vi "Main.vi"() -> ()   [LabVIEW 2015]
uses:
  <vilib>/myRIO/Instrument Drivers/Onboard IO/PWM/typedefs/PWM Reference.ctl
  <vilib>/myRIO/Common/Instrument Driver Framework/Utilities/typedefs/myRIO Generic Hardware Reference.ctl
  <vilib>/myRIO/Common/Instrument Driver Framework/Utilities/typedefs/Hardware Version Enum.ctl
  <vilib>/myRIO/Common/Instrument Driver Framework/Utilities/typedefs/myRIO v1.0 Reference.ctl
  <vilib>/myRIO/Common/Instrument Driver Framework/Utilities/typedefs/Generic FPGA Reference.ctl
  <vilib>/myRIO/Common/Instrument Driver Framework/myRIO v1.0/PWM/typedefs/PWM Channels Enum.ctl
  <vilib>/myRIO/Instrument Drivers/Onboard IO/PWM/typedefs/PWM Configuration.ctl
  <vilib>/userdefined/High Color/nirio_resource_hc.ctl
  <vilib>/myRIO/Instrument Drivers/Onboard IO/DIO/typedefs/DIO Reference.ctl
  <vilib>/myRIO/Common/Instrument Driver Framework/myRIO v1.0/DIO/typedefs/DIO Channels List.ctl
  <vilib>/myRIO/Common/Instrument Driver Framework/myRIO v1.0/DIO/typedefs/DIO Channels Enum.ctl
  <vilib>/myRIO/Common/Instrument Driver Framework/Utilities/vis/Is FPGA Ref Available.vi
  <vilib>/myRIO/Common/Instrument Driver Framework/myRIO v1.0/DIO/vis/myRIO v1.1 Open DIO.vi
  <vilib>/myRIO/Instrument Drivers/Onboard IO/DIO/vis/Write.vi
  <vilib>/myRIO/Common/Instrument Driver Framework/myRIO v1.0/PWM/vis/myRIO v1.1 Open PWM.vi
  <vilib>/myRIO/Common/Instrument Driver Framework/Utilities/vis/Validate Channels.vi
  <vilib>/myRIO/Common/Instrument Driver Framework/myRIO v1.0/DIO/vis/myRIO v1.0 Reserve DIO.vi
  <vilib>/myRIO/Common/Instrument Driver Framework/myRIO v1.0/PWM/vis/myRIO v1.0 Reserve PWM.vi
  <vilib>/myRIO/Instrument Drivers/Onboard IO/PWM/vis/Set Duty Cycle and Frequency.vi
  <vilib>/myRIO/Common/Instrument Driver Framework/myRIO v1.0/PWM/vis/myRIO v1.0 Close PWM.vi
  <vilib>/myRIO/Common/Instrument Driver Framework/myRIO v1.0/UART/vis/myRIO v1.0 Close UART.vi
  <vilib>/myRIO/Common/Instrument Driver Framework/myRIO v1.0/Resource Manager/vis/myRIO v1.0 Reserve Channel List.vi
  <vilib>/myRIO/Common/Instrument Driver Framework/myRIO v1.0/DIO/vis/myRIO v1.0 Build MUX Configuration DIO.vi
  <vilib>/myRIO/Common/Instrument Driver Framework/myRIO v1.0/PWM/vis/myRIO v1.0 Build MUX Configuration PWM.vi
  <vilib>/myRIO/Common/Instrument Driver Framework/myRIO v1.0/PWM/vis/myRIO v1.0 Unreserve PWM.vi
  <vilib>/myRIO/Common/Instrument Driver Framework/myRIO v1.0/Resource Manager/vis/myRIO v1.0 Reserve Channel.vi
  <vilib>/myRIO/Common/Instrument Driver Framework/myRIO v1.0/Resource Manager/vis/myRIO v1.0 Unreserve Channel.vi
  <vilib>/myRIO/Common/Instrument Driver Framework/myRIO v1.0/Resource Manager/vis/myRIO v1.0 Create Configuration List.vi
  <vilib>/myRIO/Common/Instrument Driver Framework/myRIO v1.0/Resource Manager/vis/myRIO v1.0 Unreserve Channel List.vi
  <vilib>/myRIO/Common/Instrument Driver Framework/myRIO v1.0/Resource Manager/vis/myRIO v1.0 Build Mutex Name.vi
  <vilib>/Utility/VariantDataType/GetNumericInfo.vi
  <vilib>/Utility/error.llb/Error Cluster From Error Code.vi
  <vilib>/myRIO/Common/Instrument Driver Framework/myRIO v1.0/myRIO v1.1 Open.vi
  <vilib>/myRIO/Common/Instrument Driver Framework/Utilities/vis/IO Manager.vi
  <vilib>/myRIO/Common/Instrument Driver Framework/Utilities/vis/Configuration Manager.vi
  <vilib>/myRIO/Common/Instrument Driver Framework/myRIO v1.0/Resource Manager/vis/myRIO v1.0 Configure IO.vi
  <vilib>/myRIO/Common/Instrument Driver Framework/myRIO v1.0/myRIO v1.0 Close.vi
  <vilib>/myRIO/Common/Instrument Driver Framework/myRIO v1.0/PWM/vis/myRIO v1.0 Write PWM.vi
  <vilib>/myRIO/Common/Instrument Driver Framework/myRIO v1.0/PWM/vis/myRIO v1.0 Shutdown PWM.vi
  <vilib>/myRIO/Common/Instrument Driver Framework/Utilities/vis/FPGA Ref Manager.vi
  <vilib>/myRIO/Common/Instrument Driver Framework/myRIO v1.0/myRIO v1.0 Reset FPGA.vi
  <vilib>/myRIO/Common/Instrument Driver Framework/myRIO v1.0/IRQ/vis/myRIO v1.0 IRQ Info FGV.vi
  <vilib>/myRIO/Common/Instrument Driver Framework/myRIO v1.0/IRQ/vis/myRIO v1.0 Timer IRQ Info FGV.vi
  <vilib>/myRIO/Common/Instrument Driver Framework/myRIO v1.0/IRQ/vis/myRIO v1.0 ISR Agent.vi
  <vilib>/myRIO/Common/Instrument Driver Framework/myRIO v1.0/DIO/vis/myRIO v1.0 Write DIO.vi
  <vilib>/myRIO/Instrument Drivers/Onboard IO/PWM/vis/myRIO PWM Open.xnode
  <vilib>/myRIO/Express VI/Onboard Devices/LED/LED Express VI.xnode
  <vilib>/myRIO/Instrument Drivers/Onboard IO/DIO/vis/myRIO DIO Open.xnode
  <vilib>/myRIO/Instrument Drivers/Onboard IO/PWM/PWM.lvlib
  <vilib>/myRIO/Instrument Drivers/Utilities/Utilities.lvlib
  <vilib>/myRIO/Instrument Drivers/Onboard IO/DIO/DIO.lvlib
panel:
  in  "Water Spill Guard":bool
  out "Sensor Pin":T1
  out "Gripper Pin":T1
  out "Pour Pin":T1
  in  "Pour":bool
  out "Information":string="Pour"
  out "Counter":dbl=1.0
  out "New Duty Cycle":dbl=nan
  in  "Stop [ESC]":bool
  in  "Gripper":bool
  out "Water Detected":bool
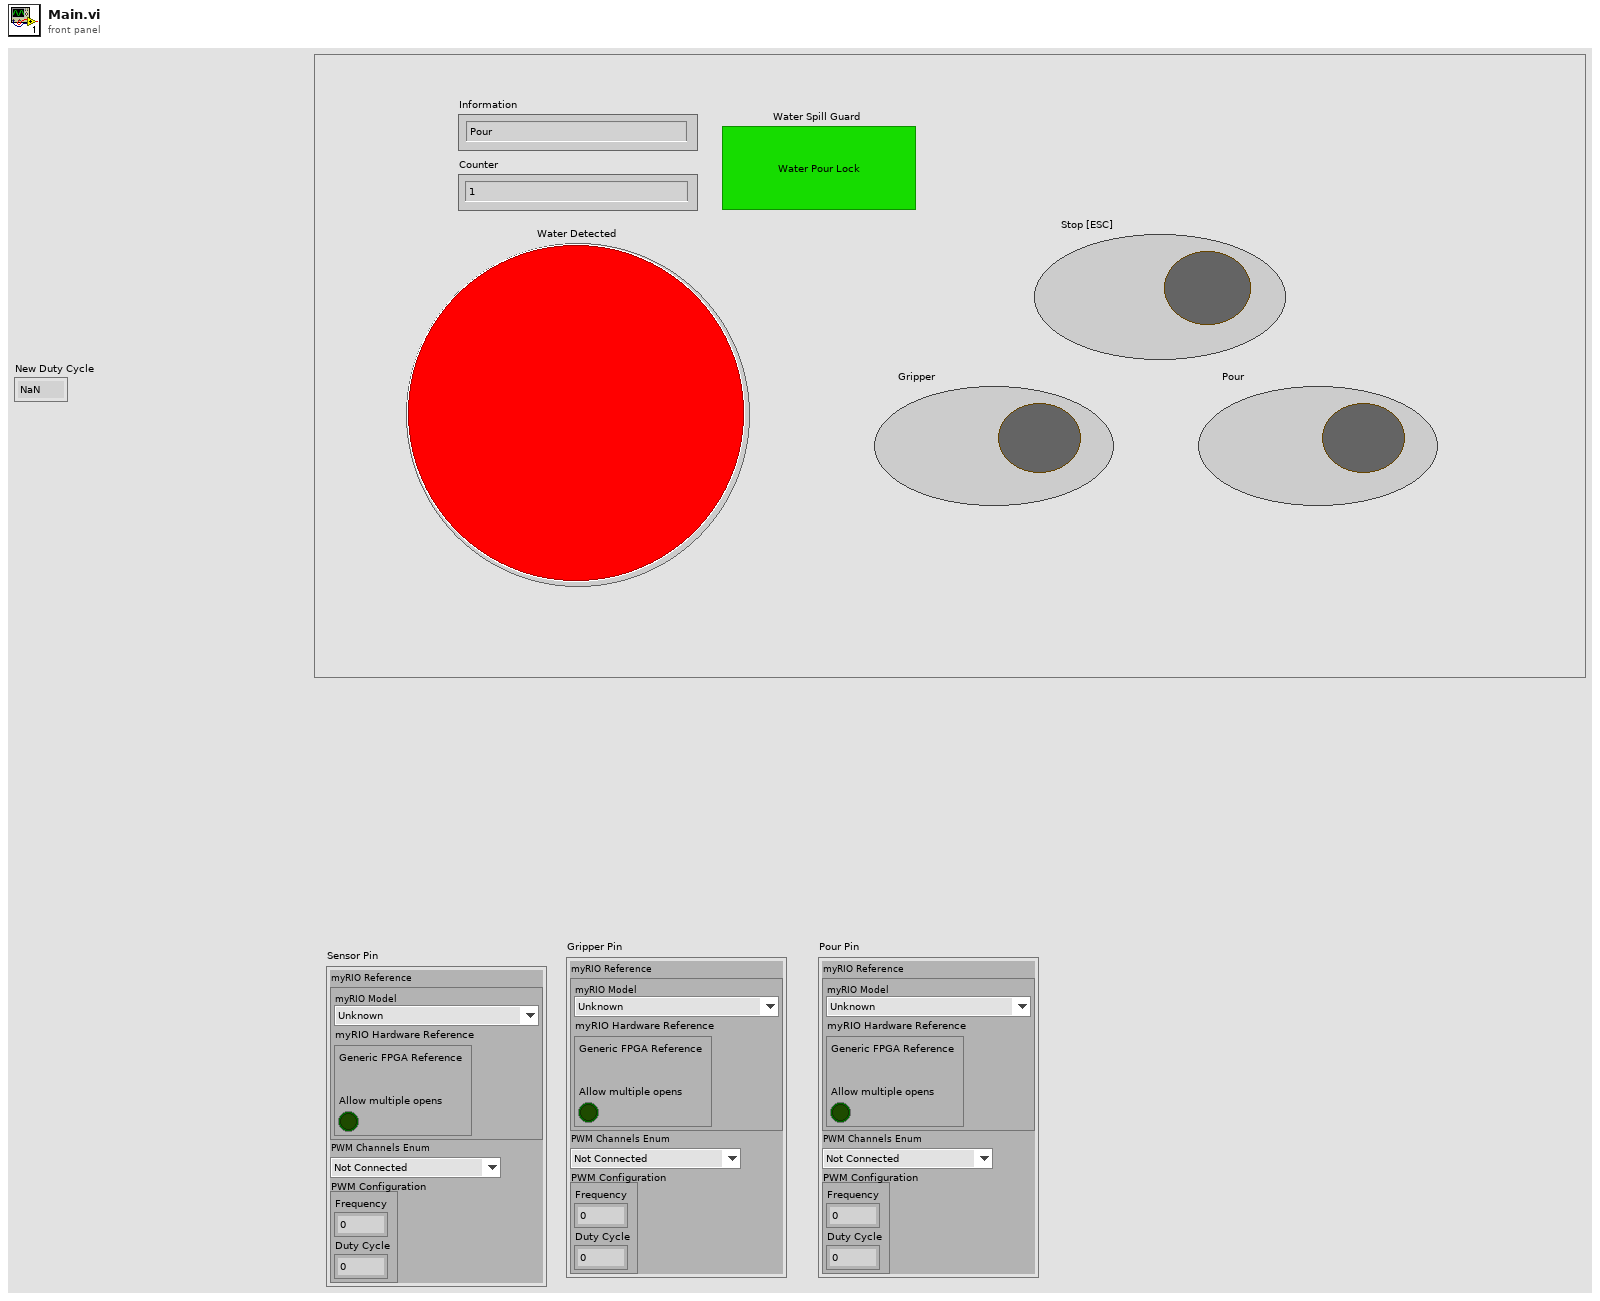
[diagram p1: front panel]
types:
  T1 = typedef "PWM.lvlib/PWM Reference.ctl" = cluster{"myRIO Reference":T2, "PWM Channels Enum":T6, "PWM Configuration":T7}
  T2 = typedef "myRIO Generic Hardware Reference.ctl" = cluster{"myRIO Model":T3, "myRIO Hardware Reference":T4}
  T3 = typedef "Hardware Version Enum.ctl" = enum16{"Unknown", "myRIO-1900", "myRIO-1950", "roboRIO"}
  T4 = typedef "myRIO v1.0 Reference.ctl" = cluster{"Generic FPGA Reference":T5, "Allow multiple opens":bool}
  T5 = typedef "Generic FPGA Reference.ctl" = refnum<k20>
  T6 = typedef "PWM Channels Enum.ctl" = enum16{"Not Connected", "C/PWM0", "C/PWM1", "A/PWM0", "A/PWM1", "A/PWM2", "B/PWM0", "B/PWM1", "B/PWM2", "PWM/PWM0", "PWM/PWM1", "PWM/PWM2", "PWM/PWM3", "PWM/PWM4", "PWM/PWM5", "PWM/PWM6", "PWM/PWM7", "PWM/PWM8", "PWM/PWM9"}
  T7 = typedef "PWM.lvlib/PWM Configuration.ctl" = cluster{"Frequency":dbl, "Duty Cycle":dbl}
  T8 = typedef "nirio_resource_hc.ctl" = tag
  T9 = typedef "DIO.lvlib/DIO Reference.ctl" = cluster{"myRIO Reference":T2, "DIO Channels List":T10}
  T10 = typedef "DIO Channels List.ctl" = T11[]
  T11 = typedef "DIO Channels Enum.ctl" = enum16{"Not Connected", "C/DIO0", "C/DIO1", "C/DIO2", "C/DIO3", "C/DIO4", "C/DIO5", "C/DIO6", "C/DIO7", "A/DIO0", "A/DIO1", "A/DIO2", "A/DIO3", "A/DIO4", "A/DIO5", "A/DIO6", "A/DIO7", "A/DIO8", "A/DIO9", "A/DIO10", "A/DIO11", "A/DIO12", "A/DIO13", "A/DIO14", "A/DIO15", "B/DIO0", "B/DIO1", "B/DIO2", "B/DIO3", "B/DIO4", "B/DIO5", "B/DIO6", "B/DIO7", "B/DIO8", "B/DIO9", "B/DIO10", "B/DIO11", "B/DIO12", "B/DIO13", "B/DIO14", "B/DIO15", "LED0", "LED1", "LED2", "LED3", "Button0", "DIO/DIO0", "DIO/DIO1", "DIO/DIO2", "DIO/DIO3", "DIO/DIO4", "DIO/DIO5", "DIO/DIO6", "DIO/DIO7", "DIO/DIO8", "DIO/DIO9", "SPI/CS0", "SPI/CS1", "SPI/CS2", "SPI/CS3", "LED RADIO (Green)", "LED RADIO (Red)", "LED COMM (Green)", "LED COMM (Red)", "LED MODE (Green)", "LED MODE (Red)"}
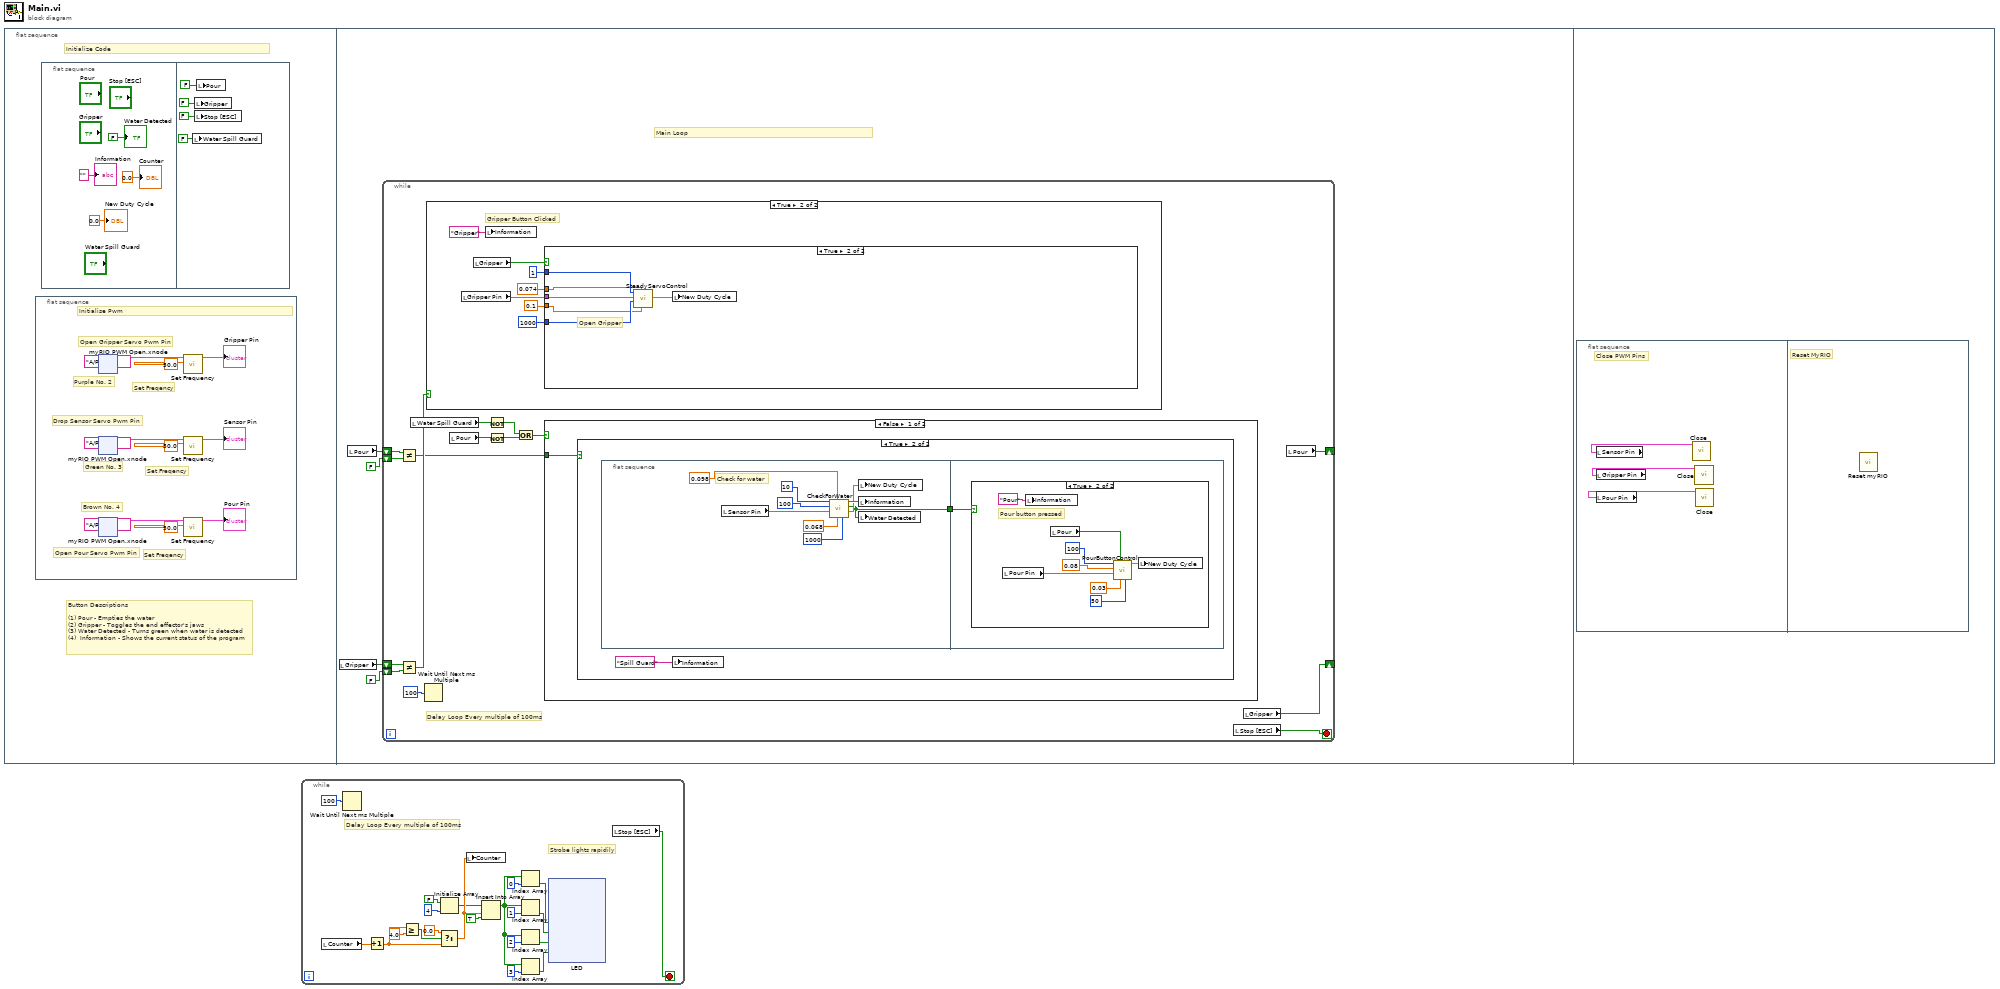
[diagram p0: block diagram]
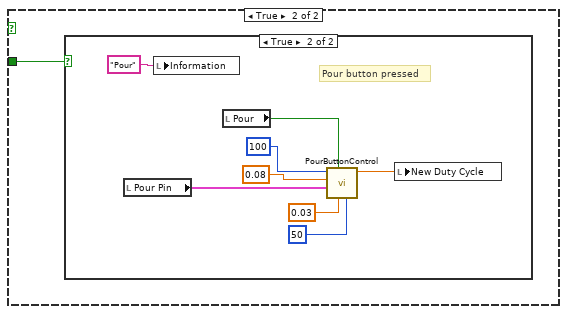
[diagram p4: hidden frame]
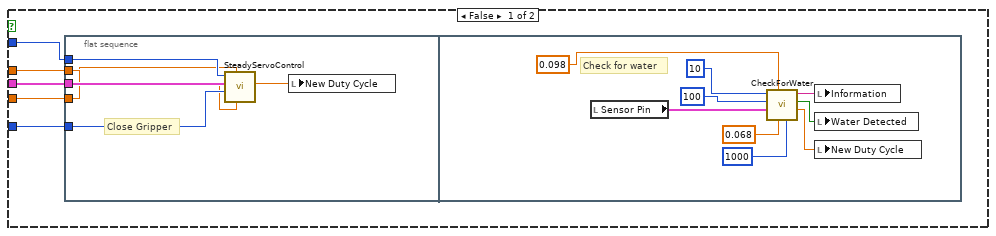
[diagram p7: hidden frame]
diagram:
  n1 = flat-sequence {
    frame #0 {
      # "Button Descriptions\n\n(1) Pour - Empties the water\n(2) Gripper - Toggles the end effector's jaws\n(3) Water Detected - Turns green when water is detected\n(4)  Information - Shows the current status of the program"
      # "Initialize Code"
      n2 = flat-sequence {
        frame #0 {
          # "Green No. 3"
          # "Set Freqency"
          # "Drop Sensor Servo Pwm Pin"
          # "Initialise Pwm"
          # "Purple No. 2"
          # "Set Freqency"
          # "Open Gripper Servo Pwm Pin"
          # "Set Freqency"
          # "Brown No. 4"
          # "Open Pour Servo Pwm Pin"
          n3 = xnode "myRIO PWM Open.xnode"("Channel Name"=tag "A/PWM2") -> ("PWM Ref Out"=w7:T1)  [unwired: 2 in, 1 out]
          n4 = xnode "myRIO PWM Open.xnode"("Channel Name"=tag "A/PWM1") -> ("PWM Ref Out"=w2:T1)  [unwired: 2 in, 1 out]
          n5 = xnode "myRIO PWM Open.xnode"("Channel Name"=tag "A/PWM0") -> ("PWM Ref Out"=w10:T1)  [unwired: 2 in, 1 out]
          n6 = call <vilib>:"Set Frequency.vi"("Frequency [Hz]"=50.0, "PWM Ref In"=w7) -> ("PWM Ref Out"=→"Gripper Pin":T1)  [unwired: 7 in, 1 out]
          n7 = call <vilib>:"Set Frequency.vi"("Frequency [Hz]"=50.0, "PWM Ref In"=w2) -> ("PWM Ref Out"=→"Sensor Pin":T1)  [unwired: 7 in, 1 out]
          n8 = call <vilib>:"Set Frequency.vi"("Frequency [Hz]"=50.0, "PWM Ref In"=w10) -> ("PWM Ref Out"=→"Pour Pin":T1)  [unwired: 7 in, 1 out]
        }
      }
      n9 = flat-sequence {
        frame #0 {
          "Water Detected" <- FALSE ("Water Detected")
          "Counter" <- 0.0 ("Counter")
          "Information" <- "" ("Information")
          "New Duty Cycle" <- 0.0 ("New Duty Cycle")
        }
        frame #1 {
          n10 = local write "Water Spill Guard"(FALSE ("Water Spill Guard")) -> ()
          n11 = local write "Gripper"(FALSE ("Pour")) -> ()
          n12 = local write "Stop [ESC]"(FALSE ("Pour")) -> ()
          n13 = local write "Pour"(FALSE ("Pour")) -> ()
        }
      }
    }
    frame #1 {
      # "Main Loop"
      n14 = local read "Gripper"() -> (w72:bool)
      n15 = local read "Pour"() -> (w70:bool)
      n16 = while {
        shift-right: [w87] -> _
        shift-left: w72 -> [w85]
        shift-left: FALSE ("Gripper") -> [w84]
        shift-right: [w79] -> _
        shift-left: w70 -> [w81]
        shift-left: FALSE ("Pour") -> [w80]
        stop <- w83 stop-if-true
        # "Delay Loop Every multiple of 100ms"
        n17 = Not Equal?(x=w81, y=w80) -> (x != y?=w73:bool)
        n18 = Not Equal?(x=w85, y=w84) -> (x != y?=w86:bool)
        n19 = local read "Water Spill Guard"() -> (w75:bool)
        n20 = Wait Until Next ms Multiple(millisecond multiple=u32 100) -> ()  [unwired: 1 out]
        n21 = case shown="True" w86 {
          frame False {
          }
          frame True {
            # "Gripper Button Clicked"
            n22 = local read "Gripper Pin"() -> (w122:T1)
            n23 = local read "Gripper"() -> (w123:bool)
            n24 = local write "Information"("Gripper" ("Information")) -> ()
            n25 = case shown="True" w123 {
              tunnel: w122 -> [w129 w147]
              tunnel: u32 1 ("Wait Time") -> [w128 w149]
              tunnel: 1000 ("Steps") -> [w127 w148]
              tunnel: 0.074 ("Prev Duty Cycle") -> [w126 w146]
              tunnel: 0.1 ("New Duty Cycle") -> [w125 w145]
              frame False {
                n26 = flat-sequence {
                  tunnel: w129 -> [w134]
                  tunnel: w128 -> [w133]
                  tunnel: w127 -> [w132]
                  tunnel: w126 -> [w131]
                  tunnel: w125 -> [w130]
                  frame #0 {
                    # "Close Gripper"
                    n27 = call "SteadyServoControl.vi"("New Duty Cycle"=w131, "Prev Duty Cycle"=w130, "Steps"=w132, "PWM Ref Out in"=w134, "Wait Time"=w133) -> ("Numeric"=w135:dbl)  [unwired: 5 in, 1 out]
                    n28 = local write "New Duty Cycle"(w135) -> ()
                  }
                  frame #1 {
                    # "Check for water"
                    n29 = local read "Sensor Pin"() -> (w137:T1)
                    n30 = call "CheckForWater.vi"("milliseconds to wait"=u32 1000, "f"=0.068, "t"=0.098, "Sensor Pin"=w137, "Steps"=100, "Wait Time"=u32 10) -> ("Numeric"=w136:dbl, "A/DIO0 (Pin 11)"=w142:bool, "Information"=w144:string)  [unwired: 3 in]
                    n31 = local write "Information"(w144) -> ()
                    n32 = local write "Water Detected"(w142) -> ()
                    n33 = local write "New Duty Cycle"(w136) -> ()
                  }
                }
              }
              frame True {
                # "Open Gripper"
                n34 = call "SteadyServoControl.vi"("New Duty Cycle"=w145, "Prev Duty Cycle"=w146, "Steps"=w148, "PWM Ref Out in"=w147, "Wait Time"=w149) -> ("Numeric"=w150:dbl)  [unwired: 5 in, 1 out]
                n35 = local write "New Duty Cycle"(w150) -> ()
              }
            }
          }
        }
        n36 = local read "Pour"() -> (w78:bool)
        n37 = Not(x=w75) -> (.not. x?=w74:bool)
        n38 = Not(x=w78) -> (.not. x?=w77:bool)
        n39 = Or(x=w74, y=w77) -> (x .or. y?=w76:bool)
        n40 = case shown="False" w76 {
          tunnel: w73 -> [w88 w109]
          frame False {
            n41 = case shown="True" w88 {
              frame False {
              }
              frame True {
                n42 = flat-sequence {
                  tunnel: [w91] -> w89
                  tunnel: w89 -> [w100]
                  frame #0 {
                    # "Check for water"
                    n43 = local read "Sensor Pin"() -> (w94:T1)
                    n44 = call "CheckForWater.vi"("milliseconds to wait"=u32 1000, "f"=0.068, "t"=0.098, "Sensor Pin"=w94, "Steps"=100, "Wait Time"=u32 10) -> ("Numeric"=w93:dbl, "A/DIO0 (Pin 11)"=w91:bool, "Information"=w99:string)  [unwired: 3 in]
                    n45 = local write "New Duty Cycle"(w93) -> ()
                    n46 = local write "Information"(w99) -> ()
                    n47 = local write "Water Detected"(w91) -> ()
                  }
                  frame #1 {
                    n48 = case shown="True" w100 {
                      frame False {
                      }
                      frame True {
                        # "Pour button pressed"
                        n49 = local read "Pour Pin"() -> (w103:T1)
                        n50 = local write "Information"("Pour" ("Information")) -> ()
                        n51 = local read "Pour"() -> (w102:bool)
                        n52 = call "PourButtonControl.vi"("Steps"=50, "Prev Duty Cycle"=0.03, "Pour"=w102, "Pour Pin"=w103, "New Duty Cycle"=0.08, "Wait Time"=u32 100) -> ("Numeric"=w108:dbl)  [unwired: 5 in]
                        n53 = local write "New Duty Cycle"(w108) -> ()
                      }
                    }
                  }
                }
                n54 = local write "Information"("Spill Guard" ("Information")) -> ()
              }
            }
          }
          frame True {
            n55 = case shown="True" w109 {
              frame False {
              }
              frame True {
                # "Pour button pressed"
                n56 = local read "Pour Pin"() -> (w115:T1)
                n57 = local write "Information"("Pour" ("Information")) -> ()
                n58 = local read "Pour"() -> (w116:bool)
                n59 = call "PourButtonControl.vi"("Steps"=50, "Prev Duty Cycle"=0.03, "Pour"=w116, "Pour Pin"=w115, "New Duty Cycle"=0.08, "Wait Time"=u32 100) -> ("Numeric"=w110:dbl)  [unwired: 5 in]
                n60 = local write "New Duty Cycle"(w110) -> ()
              }
            }
          }
        }
        n61 = local read "Stop [ESC]"() -> (w83:bool)
        n62 = local read "Gripper"() -> (w87:bool)
        n63 = local read "Pour"() -> (w79:bool)
      }
    }
    frame #2 {
      n64 = flat-sequence {
        frame #0 {
          # "Close PWM Pins"
          n65 = local read "Sensor Pin"() -> (w151:T1)
          n66 = local read "Gripper Pin"() -> (w152:T1)
          n67 = local read "Pour Pin"() -> (w153:T1)
          n68 = call <vilib>:"Close.vi"("PWM Ref In"=w151) -> ()  [unwired: 10 in, 1 out]
          n69 = call <vilib>:"Close.vi"("PWM Ref In"=w152) -> ()  [unwired: 10 in, 1 out]
          n70 = call <vilib>:"Close.vi"("PWM Ref In"=w153) -> ()  [unwired: 10 in, 1 out]
        }
        frame #1 {
          # "Reset MyRIO"
          n71 = call <vilib>:"Reset myRIO.vi"() -> ()  [unwired: 11 in, 1 out]
        }
      }
    }
  }
  n72 = while {
    stop <- w155 stop-if-true
    # "Delay Loop Every multiple of 100ms"
    # "Strobe lights rapidily"
    n73 = local read "Counter"() -> (w174:dbl)
    n74 = Wait Until Next ms Multiple(millisecond multiple=u32 100) -> ()  [unwired: 1 out]
    n75 = Increment(x=w174) -> (x+1=w159:dbl)
    n76 = Greater Or Equal?(x=w159, y=4.0) -> (x >= y?=w157:bool)
    n77 = Select(t=0.0, s=w157, f=w159) -> (s? t:f=w173:dbl)
    n78 = Initialize Array(FALSE, 4 ("dimension size")) -> (w170:bool[])
    n79 = local write "Counter"(w173) -> ()
    n80 = Insert Into Array(array=w170, index=w173, new element=TRUE ("new element/subarray")) -> (w171:bool[])
    n81 = Index Array(array=w171, index=0) -> (element=w161:bool)
    n82 = Index Array(array=w171, index=1) -> (element=w167:bool)
    n83 = Index Array(array=w171, index=2) -> (element=w168:bool)
    n84 = Index Array(array=w171, index=3) -> (element=w169:bool)
    n85 = xnode "LED"("LED0"=w161, "LED1"=w167, "LED2"=w168, "LED3"=w169) -> ()  [unwired: 1 in, 1 out]
    n86 = local read "Stop [ESC]"() -> (w155:bool)
  }
